vi "U3 Frequency Output Mode 7.vi"(10 "Timer0Value":u8=2) -> ()   [LabVIEW 2021]
panel:
  in  "TimerClockBase (U3 V1.21+)":u16(ring)=7 items=["LJ_tcSYS", "LJ_tc4MHZ", "LJ_tc12MHZ", "LJ_tc48MHZ", "LJ_tc1MHZ_DIV", "LJ_tc4MHZ_DIV", "LJ_tc12MHZ_DIV", "LJ_tc48MHZ_DIV"]
  in  "Timer/Counter Pin Offset":u8=4
  in  "FirstFound":bool=TRUE
  in  "Address":string="1"
  in  "TimerClockDivisor":u8=24
  out "Error Message":string
  # "Demonstrates 1 timer set to Frequency Output Mode 7."
  # "This VI passes a timer\nbase clock constant that\nis valid for hardware V1.21+.\nFor hardware V1.20 changes\nmust be made."
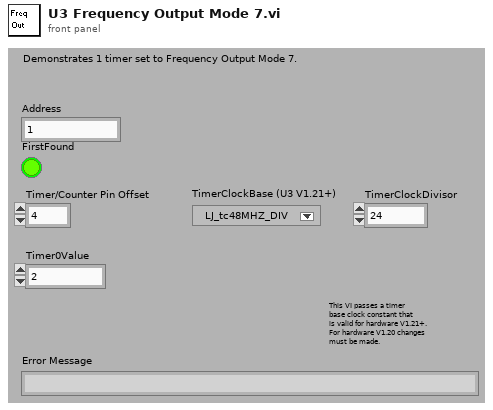
[diagram p1: front panel]
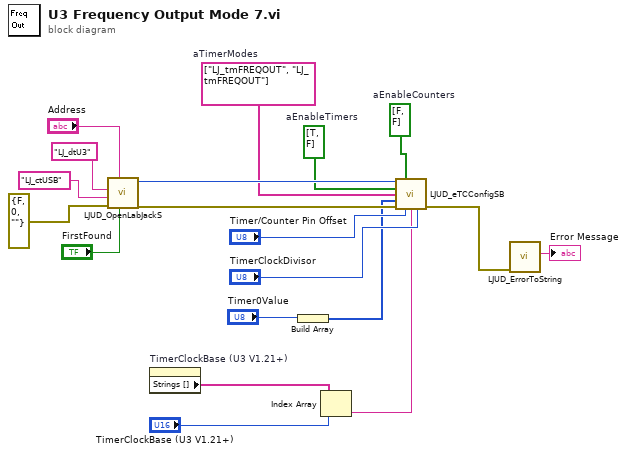
[diagram p0: block diagram]
diagram:
  w4 = bool[] [FALSE, FALSE]  # aEnableCounters
  w10 = bool[] [TRUE, FALSE]  # aEnableTimers
  w12 = string[] ["LJ_tmFREQOUT", "LJ_tmFREQOUT"]  # aTimerModes
  n1 = call "LJUD_OpenLabJackS.vi"("FirstFound"="FirstFound", "Address"="Address", "error in"=errorcluster {"status"=FALSE, "code"=0, "source"=""}, "ConnectionType"="LJ_ctUSB", "DeviceType"="LJ_dtU3") -> ("error out"=w13:errorcluster, "Handle"=w14:i32)  [unwired: 4 in, 1 out]
  n2 = property on="TimerClockBase (U3 V1.21+)" class="Ring (strict)"() -> ("Strings []"=w3:string[])  [unwired: 2 in, 2 out]
  n3 = Build Array("Timer0Value") -> (w6:u8[])
  n4 = Index Array(array=w3, index="TimerClockBase (U3 V1.21+)") -> (element=w1:string)
  n5 = call "LJUD_eTCConfigSB.vi"("Handle In"=w14, "aEnableCounters"=w4, "aEnableTimers"=w10, "aTimerModes"=w12, "aTimerValues"=w6, "error in"=w13, "TCPinOffset"="Timer/Counter Pin Offset", "TimerClockBase"=w1, "TimerClockDivisor"="TimerClockDivisor") -> ("error out"=w5:errorcluster)  [unwired: 5 in, 1 out]
  n6 = call "LJUD_ErrorToString.vi"("error in"=w5) -> ("String"=→"Error Message":string)  [unwired: 10 in]
